vi "Example.vi"() -> ()   [LabVIEW 2020]
doc: "Simple example of file operations. Comments in polish language."
panel:
  out "Data out":string
  in  "Load":bool
  in  "Clear":bool
  out "Graph":dbl[](graph) caption="Obecny pomiar"
  in  "GetData":bool
  in  "SaveData":bool
  in  "stop":bool
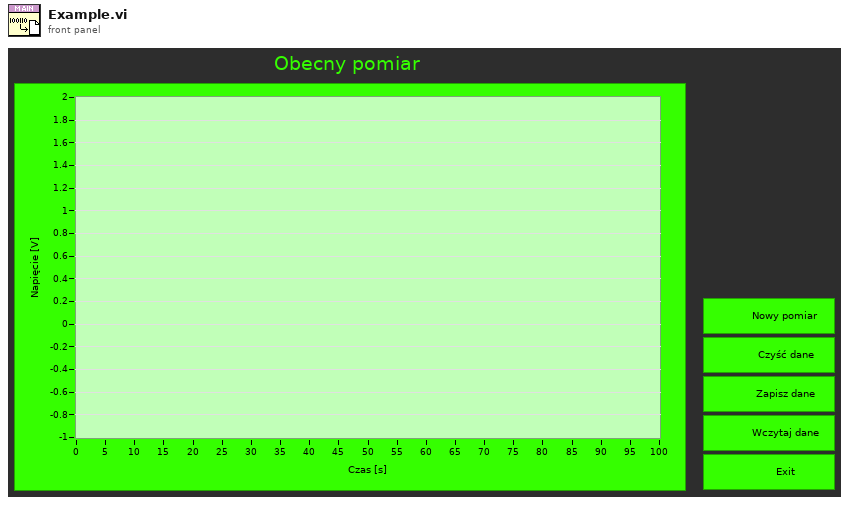
[diagram p1: front panel]
types:
  T1 = enum16{"open", "replace", "create", "open or create", "replace or create", "replace or create with confirmation"}
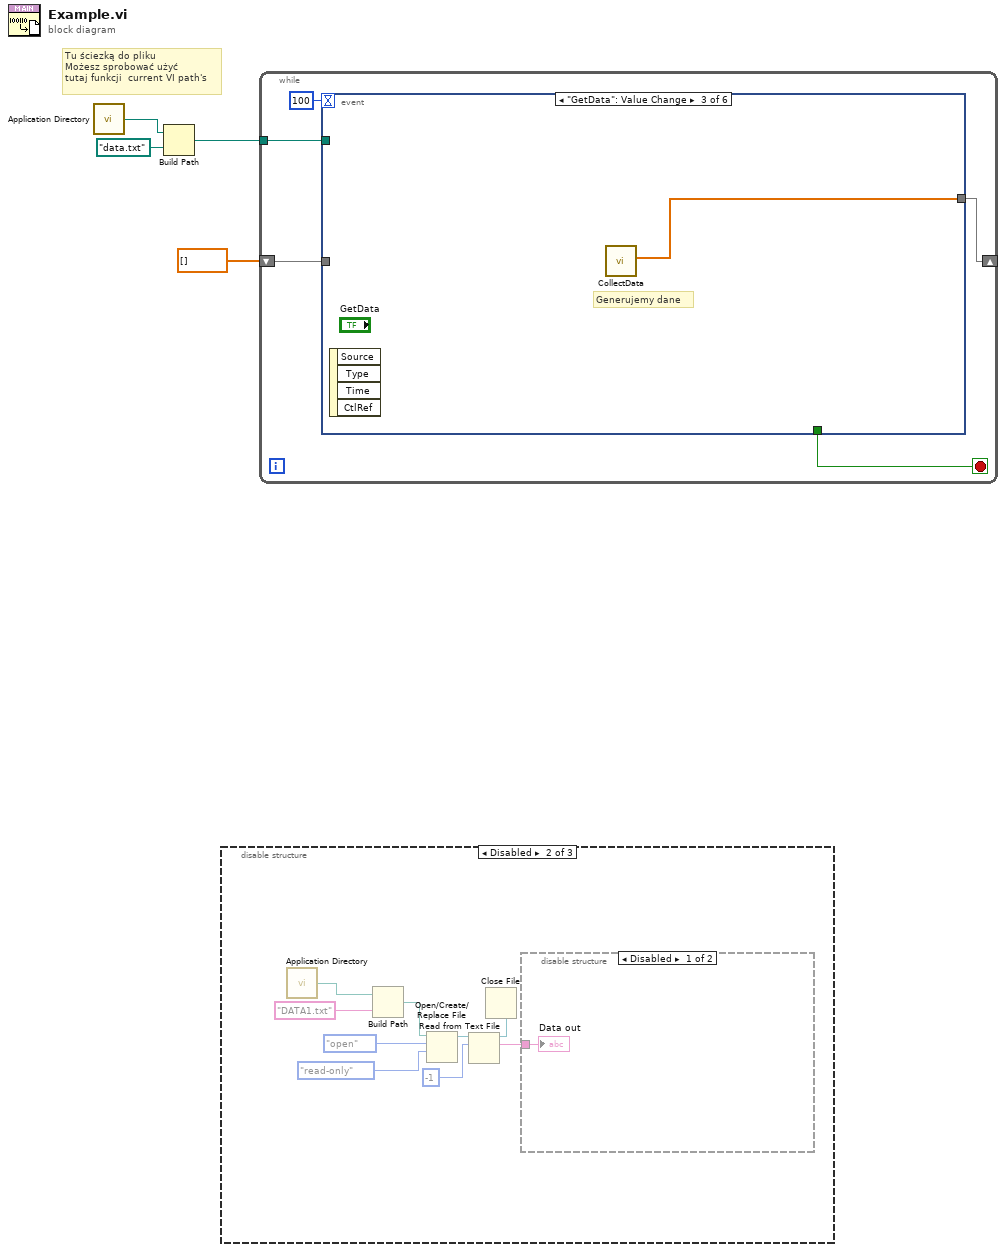
[diagram p0: block diagram]
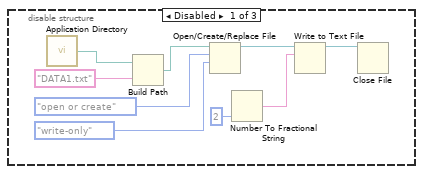
[diagram p2: hidden frame]
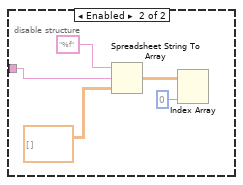
[diagram p3: hidden frame]
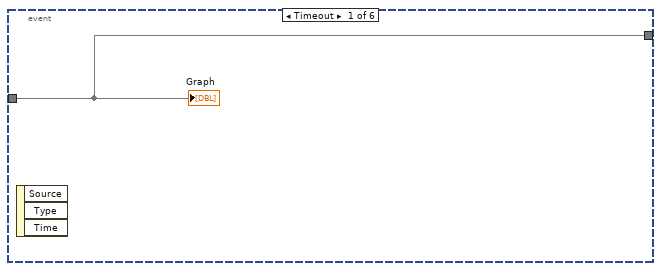
[diagram p5: hidden frame]
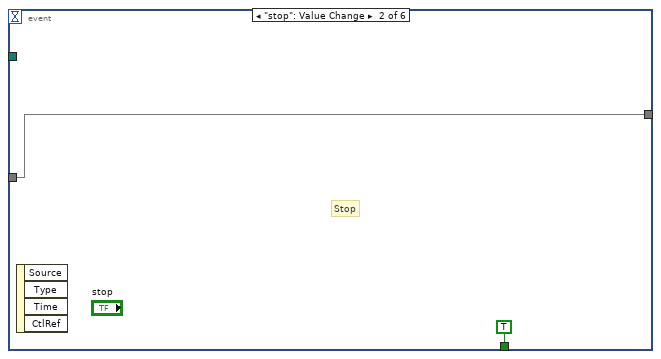
[diagram p6: hidden frame]
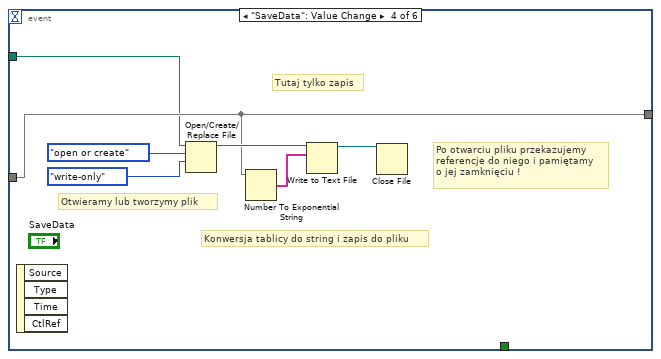
[diagram p7: hidden frame]
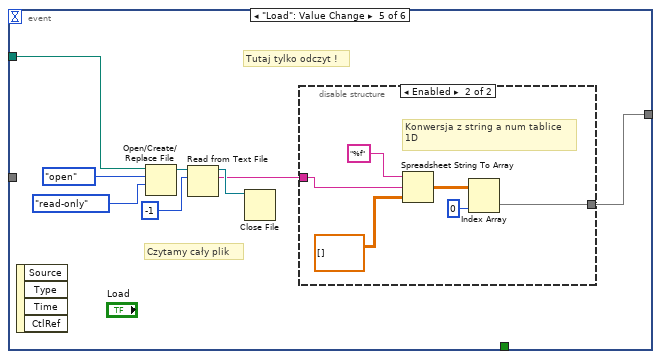
[diagram p8: hidden frame]
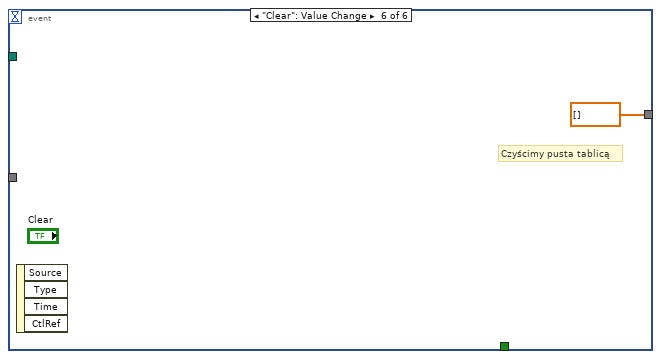
[diagram p10: hidden frame]
diagram:
  # "Tu ściezką do pliku\nMożesz sprobować użyć\ntutaj funkcji  current VI path's"
  n1 = call <vilib>:"Application Directory.vi"() -> ("Application Directory"=w3:path)
  n2 = Build Path(base path=w3, name or relative path=path "data.txt") -> (appended path=w1:path)
  n3 = disable-structure shown="Disabled" {
    frame Disabled {
      n4 = call <vilib>:"Application Directory.vi"() -> ("Application Directory"=w13:path)
      n5 = Build Path(base path=w13, name or relative path="DATA1.txt") -> (appended path=w12:path)
      n6 = Open/Create/Replace File(file path (use dialog)=w12, operation (0:open)=T1."open or create", access (0:read/write)=enum16{"read/write", "read-only", "write-only"}."write-only") -> (refnum out=w9:refnum<file>)  [unwired: 3 in, 2 out]
      n7 = Number To Fractional String(precision (6)=i16 2) -> (F-format string=w10:string)  [unwired: 3 in]
      n8 = Write to Text File(file (use dialog)=w9, text=w10) -> (refnum out=w11:refnum<file>)  [unwired: 2 in, 2 out]
      n9 = Close File(refnum=w11) -> ()  [unwired: 1 in, 2 out]
    }
    frame Disabled {
      n10 = call <vilib>:"Application Directory.vi"() -> ("Application Directory"=w21:path)
      n11 = Build Path(base path=w21, name or relative path="DATA1.txt") -> (appended path=w22:path)
      n12 = Open/Create/Replace File(file path (use dialog)=w22, operation (0:open)=T1."open", access (0:read/write)=enum16{"read/write", "read-only", "write-only"}."read-only") -> (refnum out=w20:refnum<file>)  [unwired: 3 in, 2 out]
      n13 = Read from Text File(file (use dialog)=w20, count=-1) -> (refnum out=w19:refnum<file>, text=w18:string)  [unwired: 2 in, 2 out]
      n14 = Close File(refnum=w19) -> ()  [unwired: 1 in, 2 out]
      n15 = disable-structure shown="Disabled" {
        disable-tunnel: w18 -> [w23 w29]
        frame Disabled {
          "Data out" <- w23
        }
        frame Enabled {
          n16 = Spreadsheet String To Array(format string="%f", spreadsheet string=w29, array type (2D Dbl)=dbl[][] []) -> (array=w25:dbl[][])  [unwired: 1 in]
          n17 = Index Array(array=w25, index (col)=0) -> (element=w24:dbl[])  [unwired: 1 in]
        }
      }
    }
    frame Enabled {
    }
  }
  n18 = while {
    shift-right: [w32] -> _
    shift-left: dbl[] [] -> [w33]
    tunnel: w1 -> [w30]
    stop <- w31 stop-if-true
    n19 = event shown="[2] \"GetData\": Value Change" {
      selector: _ -> [_ _ _ _ _ _]
      dyn-events: _ -> [_ _ _ _ _ _]
      timeout: 100 -> [_ _ _ _ _ _]
      tunnel: w33 -> [w35 w36 _ w42 _ _]
      tunnel: [w35 w36 w38 w42 w46 dbl[] [] ("Data")] -> w32
      tunnel: [_ TRUE ("stop") _ _ _ _] -> w31
      tunnel: w30 -> [_ _ _ w39 w47 _]
      event Timeout {
        n20 = event-data() -> ()  [unwired: 1 in, 3 out]
        "Graph" <- w35
      }
      event "stop": Value Change {
        # "Stop"
        n21 = event-data() -> ()  [unwired: 1 in, 4 out]
      }
      event "GetData": Value Change {
        # "Generujemy dane"
        n22 = event-data() -> ()  [unwired: 1 in, 4 out]
        n23 = call "CollectData.vi"() -> ("Data"=w38:dbl[])  [unwired: 6 in, 1 out]
      }
      event "SaveData": Value Change {
        # "Tutaj tylko zapis"
        # "Otwieramy lub tworzymy plik"
        # "Po otwarciu pliku przekazujemy\nreferencje do niego i pamiętamy\no jej zamknięciu !"
        # "Konwersja tablicy do string i zapis do pliku"
        n24 = event-data() -> ()  [unwired: 1 in, 4 out]
        n25 = Open/Create/Replace File(file path (use dialog)=w39, operation (0:open)=T1."open or create", access (0:read/write)=enum16{"read/write", "read-only", "write-only"}."write-only") -> (refnum out=w43:refnum<file>)  [unwired: 3 in, 2 out]
        n26 = Number To Exponential String(number=w42) -> (E-format string=w41:string[])  [unwired: 3 in]
        n27 = Write to Text File(file (use dialog)=w43, text=w41) -> (refnum out=w40:refnum<file>)  [unwired: 2 in, 2 out]
        n28 = Close File(refnum=w40) -> ()  [unwired: 1 in, 2 out]
      }
      event "Load": Value Change {
        # "Tutaj tylko odczyt !"
        # "Czytamy cały plik"
        n29 = event-data() -> ()  [unwired: 1 in, 4 out]
        n30 = Open/Create/Replace File(file path (use dialog)=w47, operation (0:open)=T1."open", access (0:read/write)=enum16{"read/write", "read-only", "write-only"}."read-only") -> (refnum out=w53:refnum<file>)  [unwired: 3 in, 2 out]
        n31 = Read from Text File(file (use dialog)=w53, count=-1) -> (refnum out=w52:refnum<file>, text=w51:string)  [unwired: 2 in, 2 out]
        n32 = Close File(refnum=w52) -> ()  [unwired: 1 in, 2 out]
        n33 = disable-structure shown="Enabled" {
          disable-tunnel: w51 -> [_ w59]
          disable-tunnel: [_ w54] -> w46
          frame Disabled {
            # "Tu surowe dane w postasci string, dodaj \nindykator  aby je podejrzeć"
          }
          frame Enabled {
            # "Konwersja z string a num tablice\n1D"
            n34 = Spreadsheet String To Array(format string="%f", spreadsheet string=w59, array type (2D Dbl)=dbl[][] []) -> (array=w55:dbl[][])  [unwired: 1 in]
            n35 = Index Array(array=w55, index (col)=0) -> (element=w54:dbl[])  [unwired: 1 in]
          }
        }
      }
      event "Clear": Value Change {
        # "Czyścimy pusta tablicą"
        n36 = event-data() -> ()  [unwired: 1 in, 4 out]
      }
    }
  }
